vi "setRefractiveIndexCompensationMode.vi"(8 "error":errorcluster, 9 "mode":i32, 10 "axis":i32, 11 "connection ID":refnum<k5>) -> (0 "error out":errorcluster, 2 "axis_out":i32, 3 "connection ID out":refnum<k5>)   [LabVIEW 2016, in "sen_api.lvlib"]
doc: "Sets the refractive index compensation mode."
uses:
  sen_api.lvlib
panel:
  out "jsonRespIn":string
  out "JSON-response":string="{\"jsonrpc\":\"2.0\",\"method\":\"\",\"params\":[5,1.245,true,\"name\"],\"id\":\"1\"}"
  out "JSON request":string
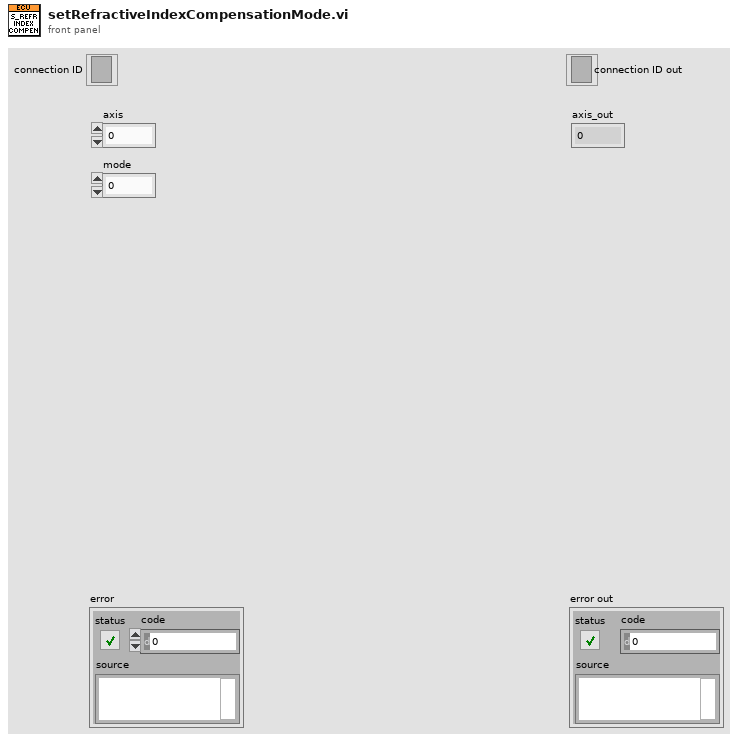
[diagram p1: front panel]
types:
  T1 = cluster{"jsonrpc":string, "method":string, "params":string[], "id":string, "api":i32, "pid":string}
  T2 = enum16{"Standard", "Buffered", "CRLF", "Immediate"}
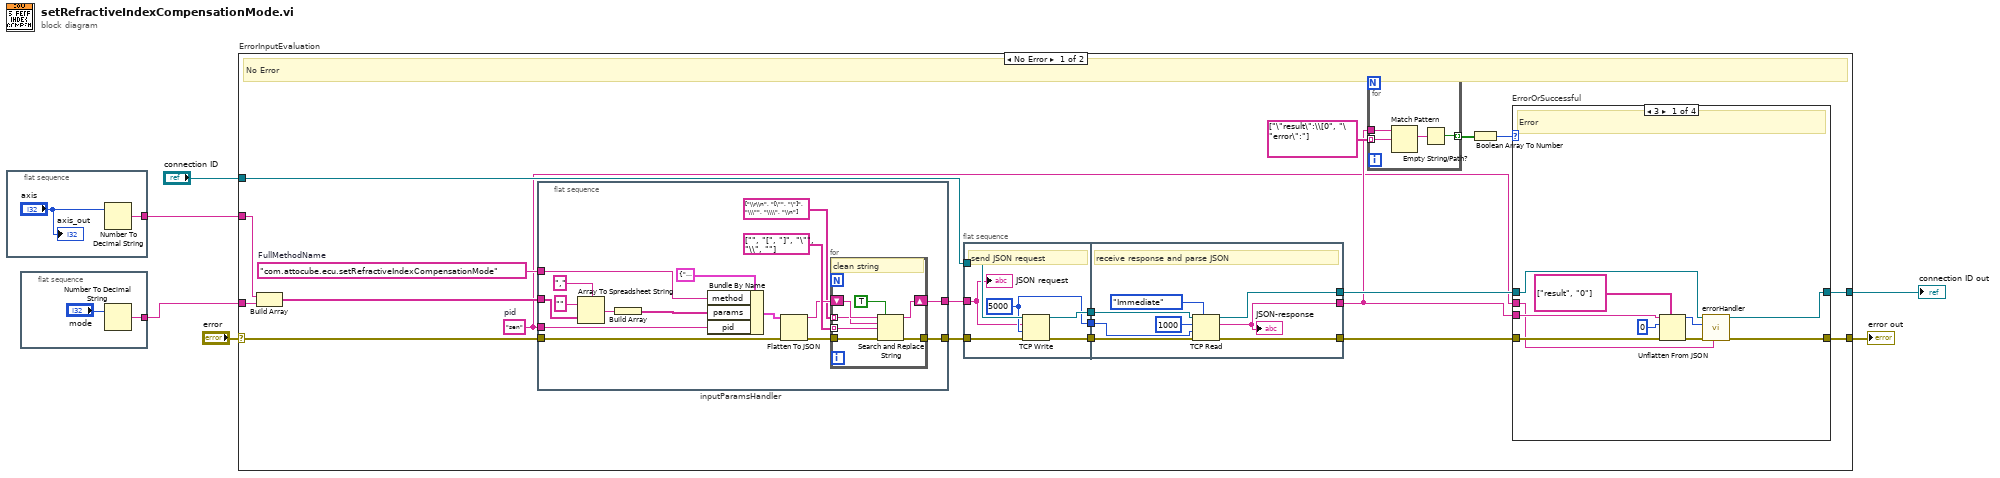
[diagram p0: block diagram]
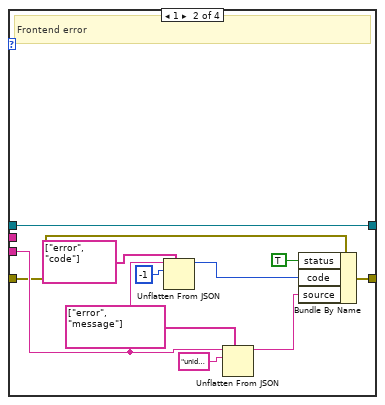
[diagram p2: hidden frame]
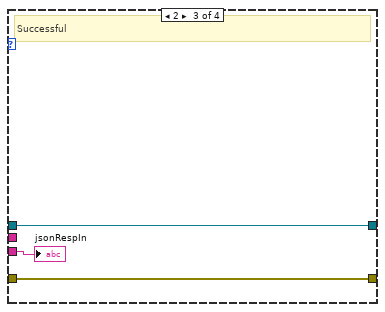
[diagram p3: hidden frame]
diagram:
  n1 = flat-sequence "in_axis" {
    tunnel: [w8] -> w2
    frame #0 {
      n2 = Number To Decimal String(number="axis") -> (decimal integer string=w8:string)  [unwired: 1 in]
      "axis_out" <- "axis"
    }
  }
  n3 = flat-sequence "in_integer" {
    tunnel: [w9] -> w1
    frame #0 {
      n4 = Number To Decimal String(number="mode") -> (decimal integer string=w9:string)  [unwired: 1 in]
    }
  }
  n5 = case "ErrorInputEvaluation" shown="No Error" "error" {
    selector: "error" -> [w17 w98]
    tunnel: "connection ID" -> [w27 w99]
    tunnel: [w19 w98] -> w5
    tunnel: [w20 w99] -> w4
    tunnel: w2 -> [w12 _]
    tunnel: w1 -> [w11 _]
    frame No Error {
      w13 = "sen"  # pid
      w18 = "com.attocube.ecu.setRefractiveIndexCompensationMode"  # FullMethodName
      # "No Error"
      n6 = Build Array ("ParametersArrayString")(w12, w11) -> (w16:string[])
      n7 = flat-sequence "inputParamsHandler" {
        tunnel: [w34] -> w15
        tunnel: w16 -> [w41]
        tunnel: w17 -> [w39]
        tunnel: [w36] -> w14
        tunnel: w18 -> [w42]
        tunnel: w13 -> [w31]
        frame #0 {
          n8 = Array To Spreadsheet String(delimiter (Tab)=",", array=w41, 3:"" ("format string")) -> (spreadsheet string=w44:string)
          n9 = Build Array "Build Array"(w44) -> (w40:string[])
          n10 = Bundle By Name(cluster=T1 {"jsonrpc"="2.0", "method"="com.attocube.amc.res.setRESReadOutFreq", "params"=[], "id"="1", "api"=2, "pid"=""}, "method"=w42, "params"=w40, "pid"=w31) -> (w43:T1)
          n11 = Flatten To JSON(anything=w43, error in (no error)=w39) -> (JSON string=w35:string, 11:w37:errorcluster)  [unwired: 1 in]
          n12 = for {
            tunnel: string[] ["\\r\\n", "[\"", "\"]", "\\\"", "\\\\", "\\n"] ("search string") -> [w50] mode=indexing
            tunnel: string[] ["", "[", "]", "\"", "\\", ""] ("replace string (\"\")") -> [w49] mode=indexing
            shift-right: [w52] -> w34
            shift-left: w35 -> [w51]
            tunnel: w37 -> [w48]
            tunnel: [w47] -> w36
            # "clean string"
            n13 = Search and Replace String(replace all?=TRUE ("replace all? (F)"), input string=w51, search string=w50, replace string=w49, error in=w48) -> (result string=w52:string, error out=w47:errorcluster)  [unwired: 3 in, 2 out]
          }
        }
      }
      n14 = flat-sequence {
        tunnel: w27 -> [w89]
        tunnel: [w87] -> w30
        tunnel: [w88] -> w29
        tunnel: w14 -> [w84]
        tunnel: [w86] -> w28
        tunnel: w15 -> [w85]
        tunnel: [w93] -> w23
        tunnel: w30 -> [w95]
        tunnel: w29 -> [w94]
        tunnel: [w91] -> w22
        tunnel: w28 -> [w92]
        tunnel: [w90] -> w21
        frame #0 {
          w86 = 5000 ("timeout ms (25000)")
          # "send JSON request"
          n15 = TCP Write(connection ID=w89, data in=w85, error in (no error)=w84, 9:w86) -> (connection ID out=w87:refnum<k5>, error out=w88:errorcluster)  [unwired: 1 out]
          "JSON request" <- w85
        }
        frame #1 {
          # "receive response and parse JSON"
          n16 = TCP Read(connection ID=w95, bytes to read=1000, error in (no error)=w94, 7:T2."Immediate" ("mode (standard)"), 9:w92) -> (connection ID out=w93:refnum<k5>, data out=w90:string, error out=w91:errorcluster)
          "JSON-response" <- w90
        }
      }
      n17 = for {
        tunnel: string[] ["\"result\":\\[0", "\"error\":"] ("path") -> [w56] mode=indexing
        tunnel: [w54] -> w25 mode=indexing
        tunnel: w21 -> [w57]
        n18 = Match Pattern(string=w57, regular expression=w56) -> (match substring=w55:string)  [unwired: 1 in, 3 out]
        n19 = Empty String/Path?(string/path=w55) -> (empty?=w54:bool)
      }
      n20 = Boolean Array To Number(Boolean array=w25) -> (number=w24:u32)
      n21 = case "ErrorOrSuccessful" shown="3" w24 {
        tunnel: w21 -> [w61 w70 w79 _]
        tunnel: w23 -> [w65 w68 w81 w83]
        tunnel: [w63 w68 w81 w83] -> w20
        tunnel: [w64 w71 w80 w82] -> w19
        tunnel: w22 -> [w67 w69 w80 w82]
        tunnel: w13 -> [w58 _ _ _]
        frame 3 {
          # "Error"
          n22 = Unflatten From JSON(path=string[] ["result", "0"], JSON string=w61, type and defaults=0, error in (no error)=w67) -> (value=w59:i32, error out=w66:errorcluster)  [unwired: 3 in]
          n23 = call "errorHandler.vi"("pid"=w58, "error in"=w66, "errNbr"=w59, "connection ID"=w65) -> ("error out 2"=w64:errorcluster, "connection ID out"=w63:refnum<k5>)  [unwired: 6 in]
        }
        frame 1 {
          # "Frontend error"
          n24 = Unflatten From JSON(path=string[] ["error", "code"], JSON string=w70, type and defaults=-1) -> (value=w77:i32)  [unwired: 4 in, 1 out]
          n25 = Unflatten From JSON(path=string[] ["error", "message"], JSON string=w70, type and defaults="unidentified error") -> (value=w78:string)  [unwired: 4 in, 1 out]
          n26 = Bundle By Name(cluster=w69, "status"=TRUE, "code"=w77, "source"=w78) -> (w71:errorcluster)
        }
        frame 2 {
          # "Successful"
          "jsonRespIn" <- w79
        }
        frame Default {
          # "NoResponse"
        }
      }
    }
    frame Error {
      # "Error"
    }
  }
  "error out" <- w5
  "connection ID out" <- w4
